vi "Main Analysis-Redirector.vi"(8 "Error In":errorcluster, 10 "VI reference":refnum<vi>, 11 "selected path":path) -> (0 "Error Out":errorcluster, 2 "Pressure":dbl, 3 "Filename Out":path=path "E:/LabVIEW/Data/Test Data/Subj-Austin_Trial-1_Condition-None.lvm" caption="Filename", 5 "error?":bool)   [LabVIEW 2020]
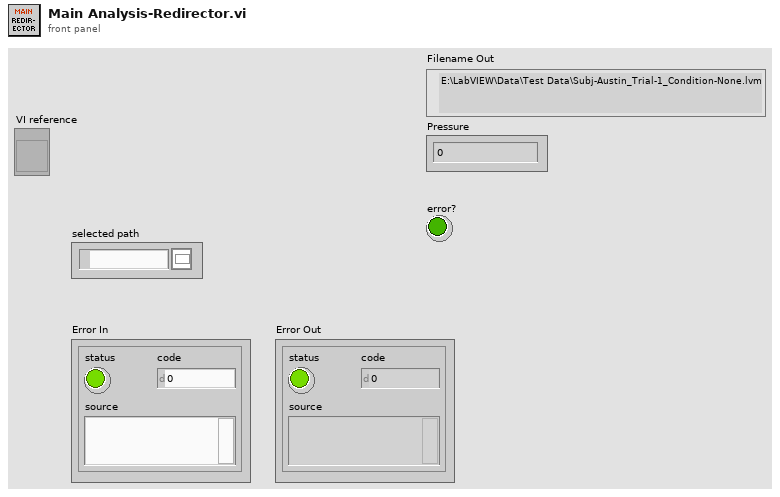
[diagram p1: front panel]
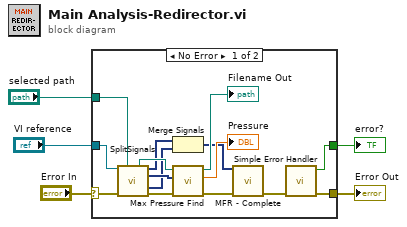
[diagram p0: block diagram]
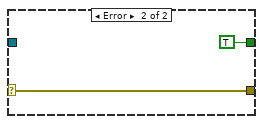
[diagram p2: hidden frame]
diagram:
  n1 = case shown="No Error" "Error In" {
    selector: "Error In" -> [w20 w22]
    tunnel: "selected path" -> [w19 _]
    tunnel: [w18 w22] -> w3
    tunnel: [w17 TRUE ("error?")] -> w2
    tunnel: "VI reference" -> [w11 _]
    frame No Error {
      n2 = call "SplitSignals.vi"("VI reference"=w11, "Filename"=w19, "Error In"=w20) -> ("Filename Out"=w15:path, "Flow"=w8:dynamicdata, "Pressure"=w14:dynamicdata, "SPL"=w7:dynamicdata, "Error Out"=w16:errorcluster)  [unwired: 5 in, 3 out]
      n3 = Merge Signals(w8, w7) -> (w6:dynamicdata)
      n4 = call "Max Pressure Find.vi"("Error In"=w16, "Pressure"=w14, "File Path"=w15) -> ("Error Out"=w10:errorcluster, "Pressure"=→"Pressure":dbl, "File Path Indicator"=→"Filename Out":path)  [unwired: 6 in]
      n5 = call "MFR - Complete.vi"("Flow, SPL & Audio"=w6, "Error In"=w10) -> ("Error Out"=w9:errorcluster)  [unwired: 9 in, 4 out]
      n6 = call <vilib>:"Simple Error Handler.vi"("error in (no error)"=w9) -> ("error?"=w17:bool, "error out"=w18:errorcluster)  [unwired: 4 in, 3 out]
    }
    frame Error {
    }
  }
  "Error Out" <- w3
  "error?" <- w2
